vi "Get All VIs in Memory Including statically-referenced Reentrant Clones_np.vi"(8 "error in (no error)":errorcluster, 11 "App Refnum":refnum<vi>) -> (0 "error out":errorcluster, 2 "All VIs in Memory Including Reentrant Clones":string[](array[string]), 3 "App Refnum Out":refnum<vi>)   [LabVIEW 2013]
panel:
  out "Number Of VIs in Memory":i32
  out "VI run time":u32
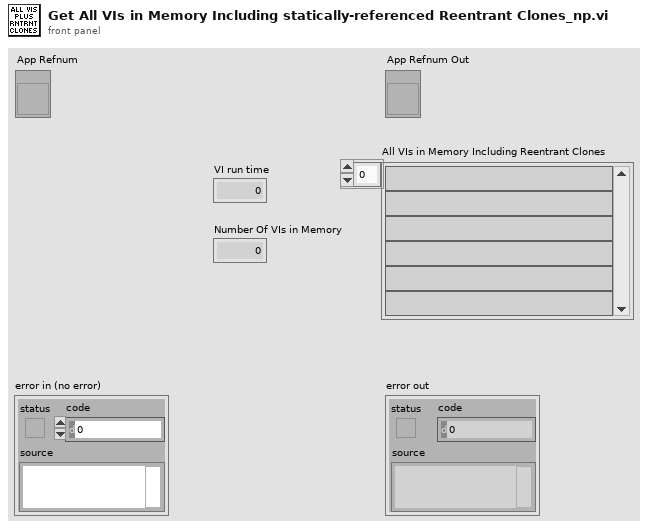
[diagram p1: front panel]
types:
  T1 = enum8{"Include the clone VI", "Include the original reentrant VI instead of the clone VI", "Include both the original reentrant VI and the clone VI"}
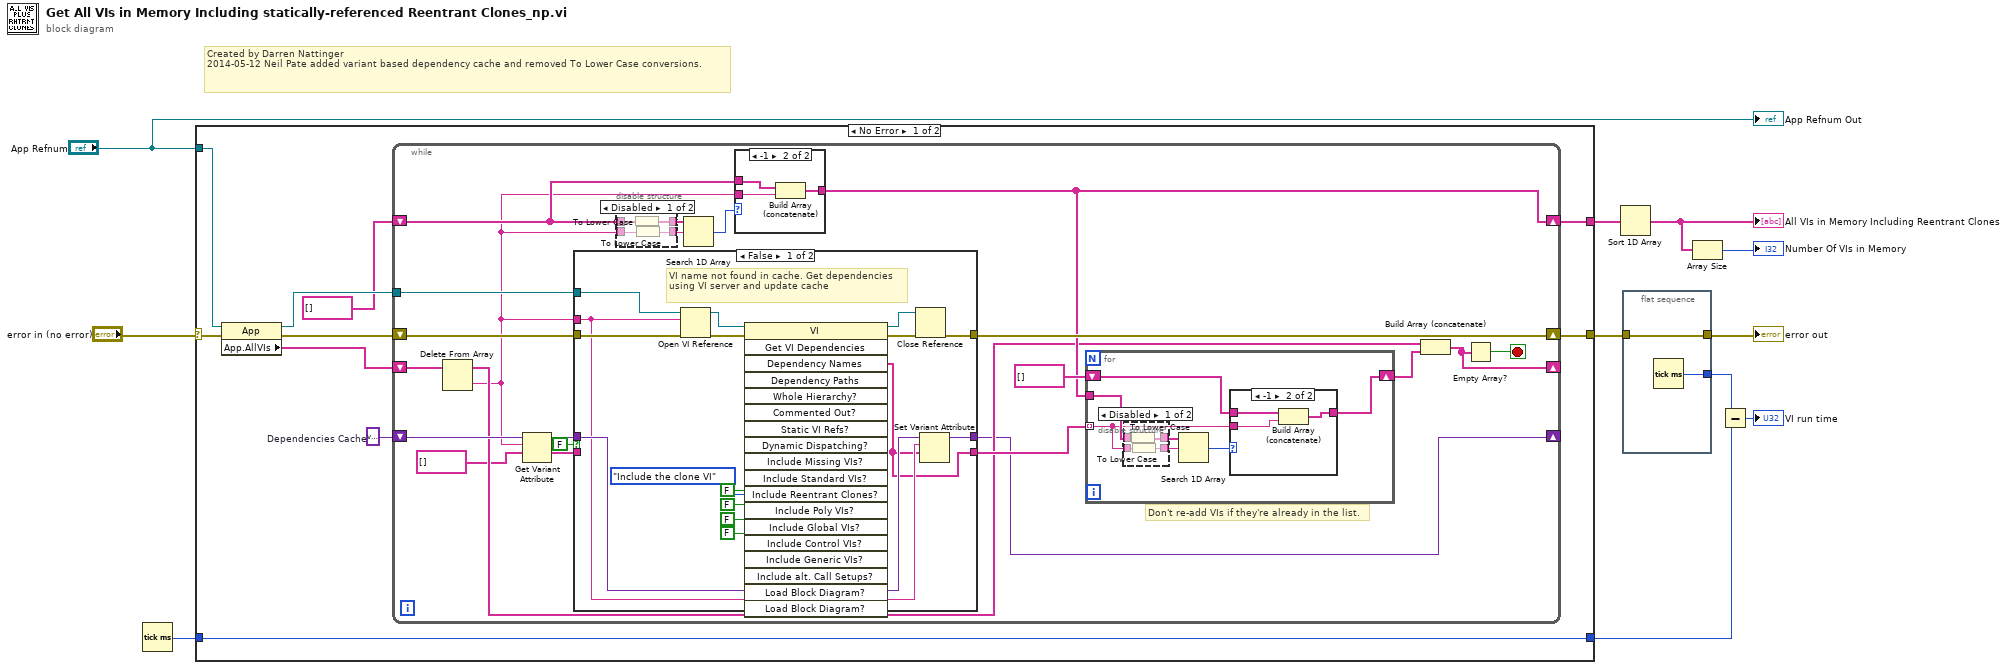
[diagram p0: block diagram]
diagram:
  # "Created by Darren Nattinger\n2014-05-12 Neil Pate added variant based dependency cache and removed To Lower Case conversions."
  n1 = Tick Count (ms)() -> (millisecond timer value=w8:u32)
  n2 = case shown="No Error" "error in (no error)" {
    selector: "error in (no error)" -> [w21 w90]
    tunnel: [w15 w90] -> w7
    tunnel: "App Refnum" -> [w14 _]
    tunnel: [w16 _] -> w10
    tunnel: w8 -> [w12 _]
    tunnel: [w12 _] -> w4
    frame No Error {
      w13 = variant  # Dependencies Cache
      n3 = property class="App"(reference=w14, error in=w21) -> (reference out=w19:refnum<vi>, error out=w20:errorcluster, "App.AllVIs"=w18:string[])
      n4 = while {
        tunnel: w19 -> [w42]
        shift-right: [w38] -> _
        shift-left: w18 -> [w40]
        shift-right: [w30] -> w16
        shift-left: string[] [] -> [w31]
        shift-right: [w39] -> w15
        shift-left: w20 -> [w43]
        shift-right: [w25] -> _
        shift-left: w13 -> [w29]
        stop <- w41 stop-if-true
        # "Don't re-add VIs if they're already in the list."
        n5 = Delete From Array(array=w40) -> (deleted portion=w27:string, array with subset deleted=w28:string[])  [unwired: 2 in]
        n6 = Get Variant Attribute(Variant=w29, name=w27, default value (empty Variant)=string[] []) -> (duplicate Variant=w26:variant, value=w24:string[])  [unwired: 1 in, 2 out]
        n7 = case shown="False" FALSE {
          tunnel: w43 -> [w65 w66]
          tunnel: w42 -> [w64 _]
          tunnel: [w54 w66] -> w39
          tunnel: [w50 w67] -> w35
          tunnel: w27 -> [w52 _]
          tunnel: w26 -> [w53 w68]
          tunnel: [w51 w68] -> w25
          tunnel: w24 -> [_ w67]
          frame False {
            # "VI name not found in cache. Get dependencies using VI server and update cache"
            n8 = Open VI Reference(application reference (local)=w64, vi path=w52, error in (no error)=w65) -> (vi reference=w63:refnum<vi>, error out=w62:errorcluster)  [unwired: 3 in]
            n9 = invoke class="VI" method="Get VI Dependencies"(reference=w63, error in=w62, "Include Reentrant Clones?"=T1."Include the clone VI", "Include Poly VIs?"=FALSE, "Include Global VIs?"=FALSE, "Include Control VIs?"=FALSE, "Include Generic VIs?"=FALSE) -> (reference out=w56:refnum<vi>, error out=w55:errorcluster, "Dependency Names"=w50:string[])  [unwired: 12 in, 16 out]
            n10 = Close Reference(reference=w56, error in (no error)=w55) -> (error out=w54:errorcluster)
            n11 = Set Variant Attribute(Variant=w53, name=w52, value=w50) -> (Variant out=w51:variant)  [unwired: 1 in, 2 out]
          }
          frame True {
            # "VI name found in cache, use dependencies from cache."
          }
        }
        n12 = disable-structure shown="Disabled" {
          disable-tunnel: [w47 w48] -> w34
          disable-tunnel: [w46 w49] -> w33
          disable-tunnel: w31 -> [w45 w49]
          disable-tunnel: w27 -> [w44 w48]
          frame Disabled {
            n13 = To Lower Case(string=w45) -> (all lower case string=w46:string[])
            n14 = To Lower Case(string=w44) -> (all lower case string=w47:string)
          }
          frame Enabled {
          }
        }
        n15 = Search 1D Array(1D array=w33, element=w34) -> (index of element=w32:i32)  [unwired: 1 in]
        n16 = case shown="-1" w32 {
          tunnel: w31 -> [w69 w72]
          tunnel: w27 -> [_ w71]
          tunnel: [w69 w70] -> w30
          frame Default {
          }
          frame -1 {
            n17 = Build Array (concatenate)(w72, w71) -> (w70:string[])
          }
        }
        n18 = for {
          tunnel: w30 -> [w79]
          tunnel: w35 -> [w73] mode=indexing
          shift-right: [w74] -> w36
          shift-left: string[] [] -> [w75]
          n19 = disable-structure shown="Disabled" {
            disable-tunnel: w79 -> [w83 w85]
            disable-tunnel: [w82 w85] -> w78
            disable-tunnel: [w81 w84] -> w77
            disable-tunnel: w73 -> [w80 w84]
            frame Disabled {
              n20 = To Lower Case(string=w83) -> (all lower case string=w82:string[])
              n21 = To Lower Case(string=w80) -> (all lower case string=w81:string)
            }
            frame Enabled {
            }
          }
          n22 = Search 1D Array(1D array=w78, element=w77) -> (index of element=w76:i32)  [unwired: 1 in]
          n23 = case shown="-1" w76 {
            tunnel: w75 -> [w86 w89]
            tunnel: [w86 w88] -> w74
            tunnel: w73 -> [_ w87]
            frame Default {
            }
            frame -1 {
              n24 = Build Array (concatenate)(w89, w87) -> (w88:string[])
            }
          }
        }
        n25 = Build Array (concatenate)(w28, w36) -> (w38:string[])
        n26 = Empty Array?(array=w38) -> (empty?=w41:bool)
      }
    }
    frame Error {
    }
  }
  n27 = Sort 1D Array(array=w10) -> (sorted array=w2:string[])
  "All VIs in Memory Including Reentrant Clones" <- w2
  n28 = flat-sequence {
    tunnel: w7 -> [w92]
    tunnel: [w92] -> w6
    tunnel: [w91] -> w5
    frame #0 {
      n29 = Tick Count (ms)() -> (millisecond timer value=w91:u32)
    }
  }
  n30 = Array Size(array=w2) -> (size(s)=→"Number Of VIs in Memory":i32)
  n31 = Subtract(x=w5, y=w4) -> (x-y=→"VI run time":u32)
  "error out" <- w6
  "App Refnum Out" <- "App Refnum"
